vi "Average strain data.vi"(8 "Error In":errorcluster, 9 "Window points":i32=5, 10 "Strain data in":T1) -> (0 "Error Out":errorcluster, 2 "Avg Strain data out":T1)   [LabVIEW 2016]
uses:
  <vilib>/ptbypt/NI_PtbyPt.lvlib
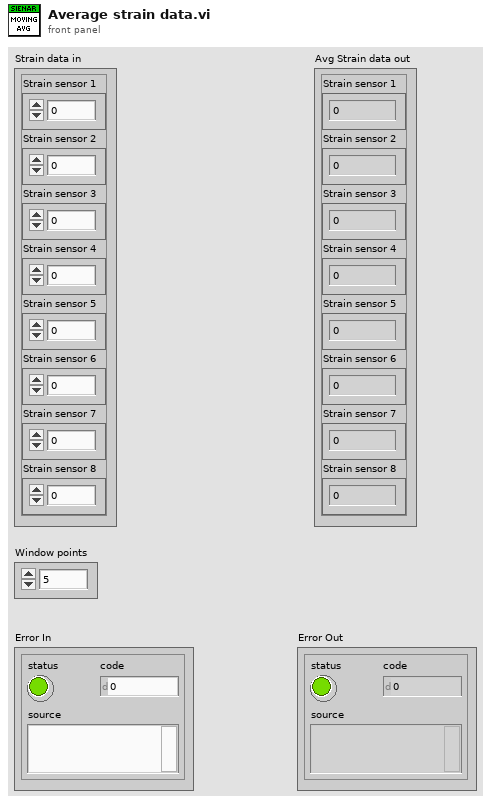
[diagram p1: front panel]
types:
  T1 = cluster{"Strain sensor 1":sgl, "Strain sensor 2":sgl, "Strain sensor 3":sgl, "Strain sensor 4":sgl, "Strain sensor 5":sgl, "Strain sensor 6":sgl, "Strain sensor 7":sgl, "Strain sensor 8":sgl}
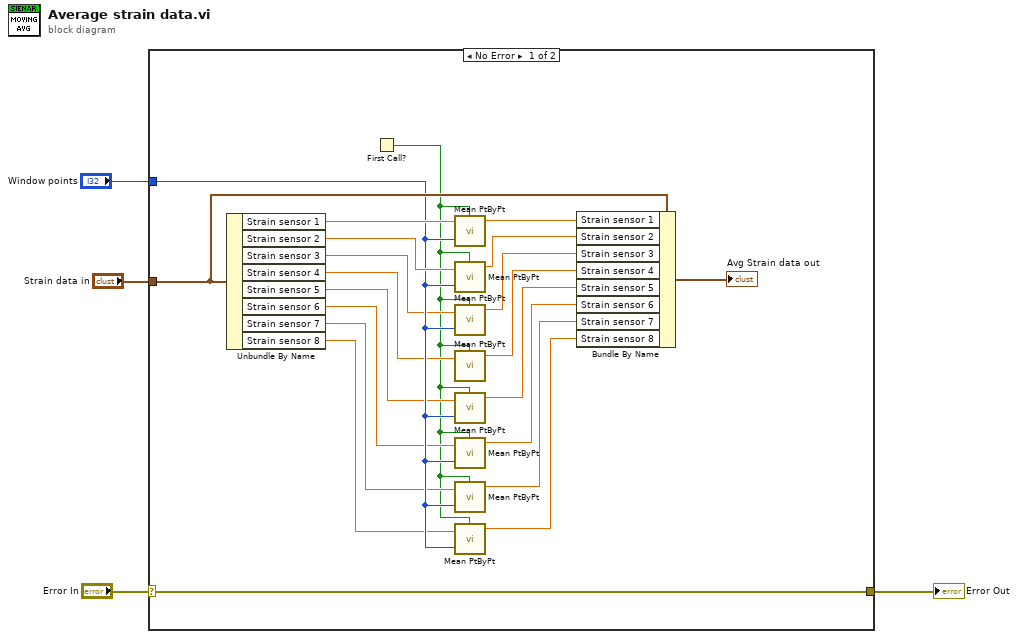
[diagram p0: block diagram]
diagram:
  n1 = case shown="No Error" "Error In" {
    selector: "Error In" -> [w25 w26]
    tunnel: [w25 w26] -> w3
    tunnel: "Strain data in" -> [w23 _]
    tunnel: "Window points" -> [w20 _]
    frame No Error {
      n2 = Unbundle By Name(w23) -> ("Strain sensor 1"=w24:sgl, "Strain sensor 2"=w21:sgl, "Strain sensor 3"=w19:sgl, "Strain sensor 4"=w18:sgl, "Strain sensor 5"=w17:sgl, "Strain sensor 6"=w16:sgl, "Strain sensor 7"=w15:sgl, "Strain sensor 8"=w14:sgl)
      n3 = First Call?() -> (First Call?: T/F=w5:bool)
      n4 = call <vilib>:"Mean PtByPt.vi"("x"=w24, "sample length"=w20, "initialize"=w5) -> ("mean"=w13:dbl)  [unwired: 1 in, 1 out]
      n5 = call <vilib>:"Mean PtByPt.vi"("x"=w21, "sample length"=w20, "initialize"=w5) -> ("mean"=w12:dbl)  [unwired: 1 in, 1 out]
      n6 = call <vilib>:"Mean PtByPt.vi"("x"=w19, "sample length"=w20, "initialize"=w5) -> ("mean"=w11:dbl)  [unwired: 1 in, 1 out]
      n7 = call <vilib>:"Mean PtByPt.vi"("x"=w18, "initialize"=w5) -> ("mean"=w10:dbl)  [unwired: 2 in, 1 out]
      n8 = call <vilib>:"Mean PtByPt.vi"("x"=w17, "sample length"=w20, "initialize"=w5) -> ("mean"=w9:dbl)  [unwired: 1 in, 1 out]
      n9 = call <vilib>:"Mean PtByPt.vi"("x"=w16, "sample length"=w20, "initialize"=w5) -> ("mean"=w8:dbl)  [unwired: 1 in, 1 out]
      n10 = call <vilib>:"Mean PtByPt.vi"("x"=w15, "sample length"=w20, "initialize"=w5) -> ("mean"=w7:dbl)  [unwired: 1 in, 1 out]
      n11 = call <vilib>:"Mean PtByPt.vi"("x"=w14, "sample length"=w20, "initialize"=w5) -> ("mean"=w6:dbl)  [unwired: 1 in, 1 out]
      n12 = Bundle By Name(cluster=w23, "Strain sensor 1"=w13, "Strain sensor 2"=w12, "Strain sensor 3"=w11, "Strain sensor 4"=w10, "Strain sensor 5"=w9, "Strain sensor 6"=w8, "Strain sensor 7"=w7, "Strain sensor 8"=w6) -> (→"Avg Strain data out":T1)
    }
    frame Error {
    }
  }
  "Error Out" <- w3
